vi "StMotor_dir_final.vi"() -> ()   [LabVIEW 2018]
doc: "This example shows how to use the Arduino Stepper Motor API. The fritzing diagram shows use with the EasyStepper 4.3 or 4.4 motor controller."
uses:
  <vilib>/LabVIEW Interface for Arduino/Type Defs/Connection Type.ctl
  <vilib>/LabVIEW Interface for Arduino/LabVIEW Interface for Arduino.lvlib
panel:
  out "stop motion 2":bool
  in  "MOTION":bool
  in  "?":i8(slide) step=2 scale=0.0..2.0
  in  "VISA resource":refnum<visa-resource-name>
  in  "Stop":bool
  in  "Stepper #":u8=1
  in  "OK Button":bool
  in  "Set Speed (Steps per second)":i16=100 min=0 max=3000 step=50
  out "Stepping?":bool
  in  "error in":errorcluster
  # "OFF"
  # "ON"
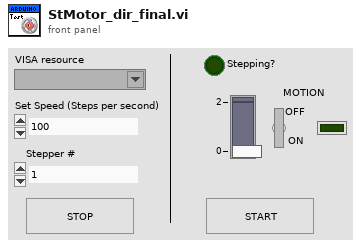
[diagram p1: front panel]
types:
  T1 = typedef "LabVIEW Interface for Arduino.lvlib/Connection Type.ctl" = enum8{"USB / Serial", "XBEE", "BlueSmirf (Bluetooth)"}
  T2 = typedef "LabVIEW Interface for Arduino.lvlib/Arduino Resource.ctl" = cluster{"VISA resource":refnum<visa-resource-name>, "Board Type":T3, "Connection Type":enum8{"USB / Serial"}, "Bytes Per Packet (15)":u8}
  T3 = typedef "LabVIEW Interface for Arduino.lvlib/Board Type.ctl" = enum16{"Uno", "Dimuelanove w/Atmega 328", "Mega 2560"}
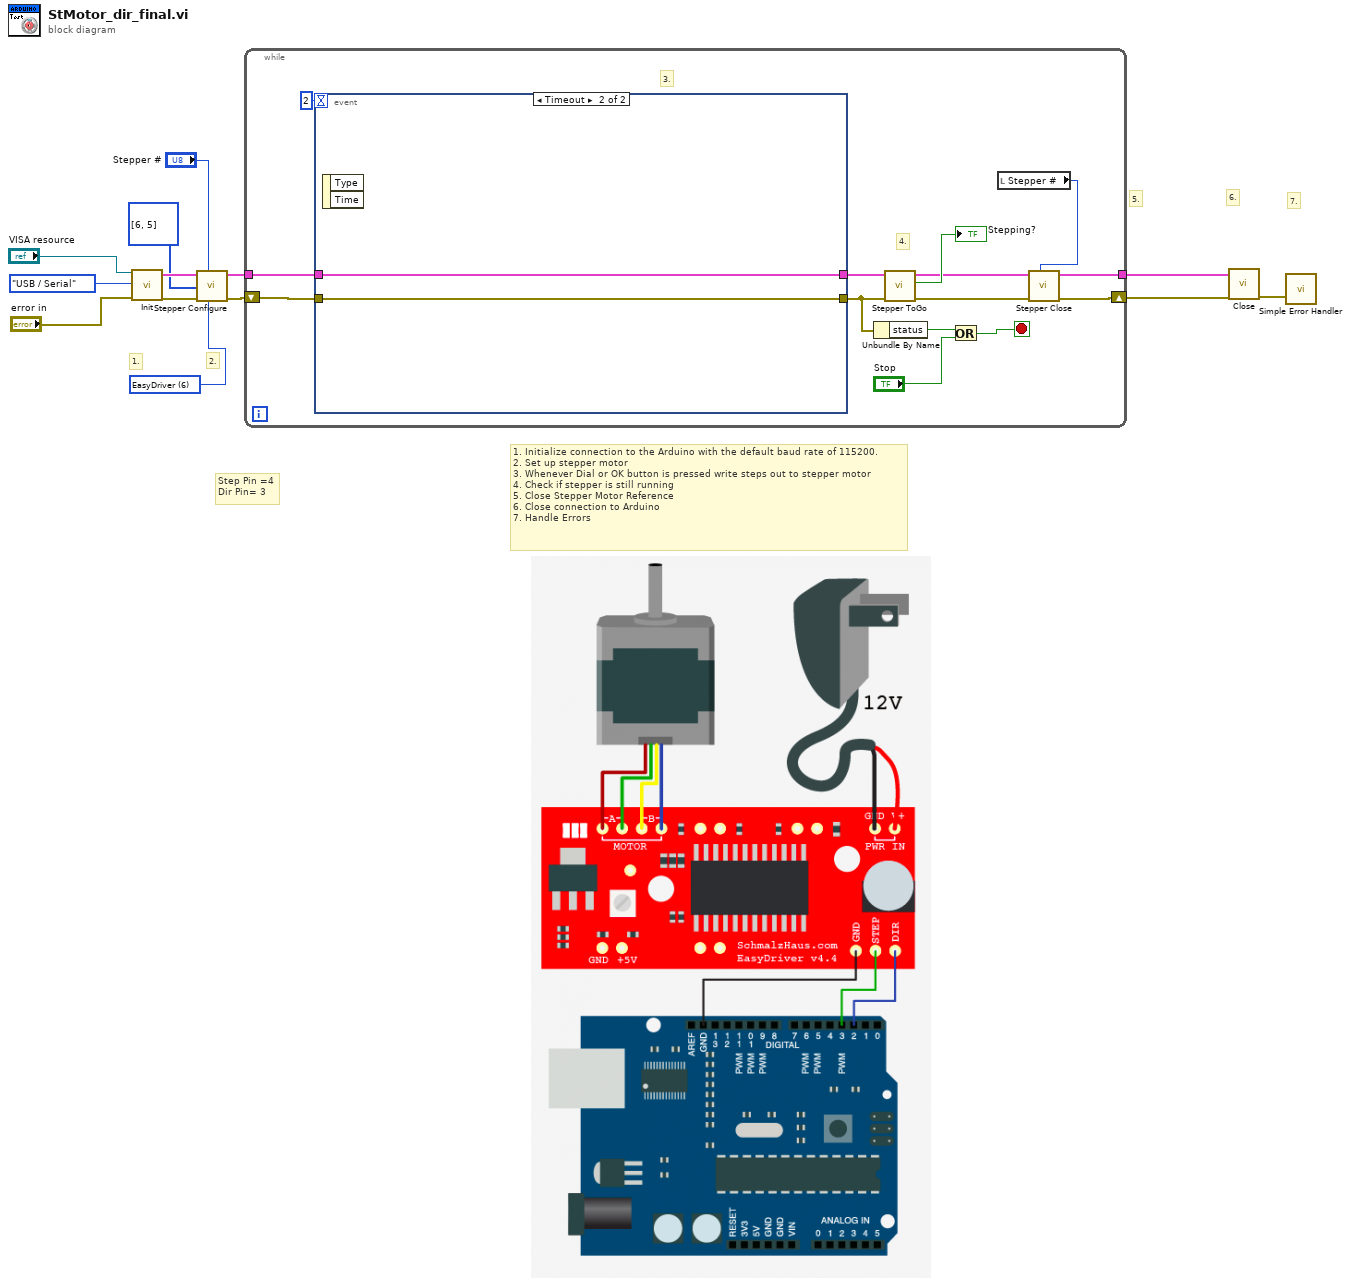
[diagram p0: block diagram]
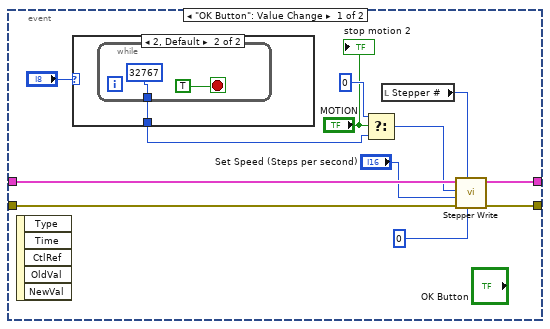
[diagram p2: hidden frame]
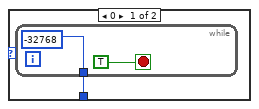
[diagram p3: hidden frame]
diagram:
  w6 = u8 6 items=["2 Wire (Pulse & Direction)"=1, "2 Wire"=2, "4 Wire"=4, "EasyDriver"=6, "AF Motor Shield (Stepper 1 & 2 Only)"=5] ("Control Method")
  # "Step Pin =4\nDir Pin= 3"
  # "7."
  # "6."
  # "5."
  # "2."
  # "1."
  # "1. Initialize connection to the Arduino with the default baud rate of 115200.\n2. Set up stepper motor\n3. Whenever Dial or OK button is pressed write steps out to stepper motor\n4. Check if stepper is still running\n5. Close Stepper Motor Reference \n6. Close connection to Arduino\n7. Handle Errors"
  n1 = call <vilib>:"Init.vi"("VISA resource"="VISA resource", "Connection Type (USB/Serial)"=Connection_Type."USB / Serial" ("Connection type"), "error in"="error in") -> ("Arduino Resource"=w9:T2, "error out"=w8:errorcluster)  [unwired: 15 in]
  n2 = call <vilib>:"Stepper Configure.vi"("Control Method"=w6, "Stepper #"="Stepper #", "error in"=w8, "Stepper Pins"=u8[] [6, 5], "Arduino Resource"=w9) -> ("error out"=w11:errorcluster, "Arduino Resource Out"=w12:T2)  [unwired: 5 in]
  n3 = while {
    tunnel: w12 -> [w26]
    shift-right: [w14] -> w1
    shift-left: w11 -> [w27]
    tunnel: [w16] -> w2
    stop <- w24 stop-if-true
    # "4."
    # "3."
    n4 = event shown="[1] Timeout" {
      selector: _ -> [_ _]
      dyn-events: _ -> [_ _]
      timeout: 2 -> [_ _]
      tunnel: w27 -> [w38 w46]
      tunnel: w26 -> [w36 w47]
      tunnel: [w37 w47] -> w22
      tunnel: [w39 w46] -> w20
      event "OK Button": Value Change {
        n5 = event-data() -> ()  [unwired: 1 in, 5 out]
        n6 = case shown="2, Default" "?" {
          tunnel: [w40 w43] -> w30
          frame 0 {
            n7 = while {
              tunnel: [i16 -32768 ("# of Steps to Move")] -> w40
              stop <- TRUE ("Stop Reverse movement") stop-if-true
            }
          }
          frame 2, Default {
            n8 = while {
              tunnel: [i16 32767 ("# of Steps to Move")] -> w43
              stop <- TRUE ("Stop Forward movement") stop-if-true
            }
          }
        }
        n9 = Select(t=0, s="MOTION", f=w30) -> (s? t:f=w29:i32)
        n10 = local read "Stepper #"() -> (w33:u8)
        n11 = call <vilib>:"Stepper Write.vi"("Set Acceleration (0 to disable)"=i16 0 ("Set acceleration"), "Stepper #"=w33, "error in"=w38, "Set Speed (Steps per Second)"="Set Speed (Steps per second)", "# of Steps to Move"=w29, "Arduino Resource"=w36) -> ("error out"=w39:errorcluster, "Arduino Resource Out"=w37:T2)  [unwired: 4 in]
        "stop motion 2" <- "MOTION"
      }
      event Timeout {
        n12 = event-data() -> ()  [unwired: 1 in, 2 out]
      }
    }
    n13 = Unbundle By Name(w20) -> ("status"=w23:bool)
    n14 = call <vilib>:"Stepper ToGo.vi"("error in"=w20, "Arduino Resource"=w22) -> ("error out"=w18:errorcluster, "Steps Remaining?"=→"Stepping?":bool, "Arduino Resource Out"=w17:T2)  [unwired: 6 in, 1 out]
    n15 = Or(x=w23, y="Stop") -> (x .or. y?=w24:bool)
    n16 = local read "Stepper #"() -> (w15:u8)
    n17 = call <vilib>:"Stepper Close.vi"("Stepper #"=w15, "error in"=w18, "Arduino Resource"=w17) -> ("error out"=w14:errorcluster, "Arduino Resource Out"=w16:T2)  [unwired: 7 in]
  }
  n18 = call <vilib>:"Close.vi"("Arduino Resource"=w2, "error in"=w1) -> ("error out"=w13:errorcluster)  [unwired: 13 in]
  n19 = call <vilib>:"Simple Error Handler.vi"("error in (no error)"=w13) -> ()  [unwired: 4 in, 5 out]
